vi "Write rotator.vi"(8 "error in (no error)":errorcluster, 10 "Rotator.lvclass":refnum<class "Rotator.lvclass">, 11 "ScienceTargetConfiguration in":refnum<class "ScienceTargetConfiguration.lvclass">) -> (0 "error out":errorcluster, 3 "ScienceTargetConfiguration out":refnum<class "ScienceTargetConfiguration.lvclass">)   [LabVIEW 2014, in "TCSDataDefinitions.lvlib" / "TCSCommand.lvlib" / "TargetConfiguration.lvlib" / "ScienceTargetConfiguration.lvclass"]
uses:
  ScienceTargetConfiguration.lvclass
  Rotator/Rotator.lvclass
  ScienceTargetConfiguration.lvclass/ScienceTargetConfiguration.ctl
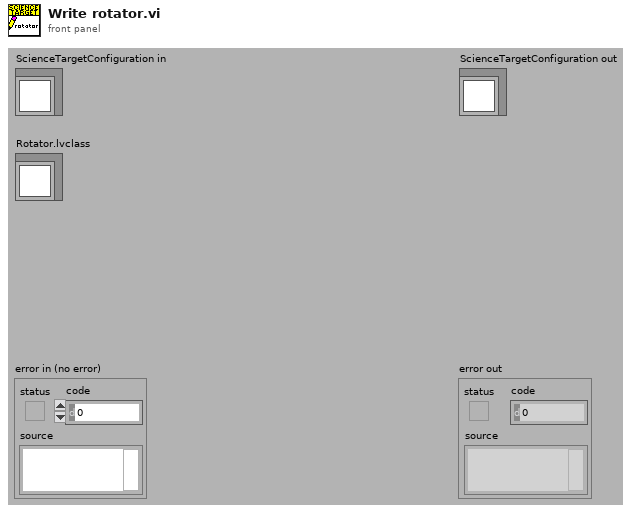
[diagram p1: front panel]
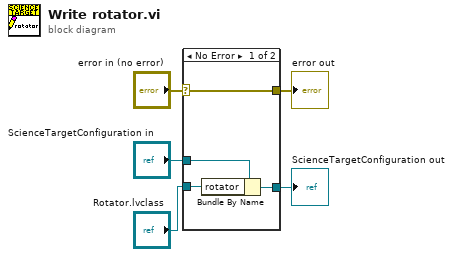
[diagram p0: block diagram]
diagram:
  n1 = case shown="No Error" "error in (no error)" {
    selector: "error in (no error)" -> [w9 w10]
    tunnel: [w9 w10] -> w4
    tunnel: [w7 w11] -> w2
    tunnel: "ScienceTargetConfiguration in" -> [w8 w11]
    tunnel: "Rotator.lvclass" -> [w6 _]
    frame No Error {
      n2 = Bundle By Name(cluster=w8, "rotator"=w6) -> (w7:refnum<class "ScienceTargetConfiguration.lvclass">)
    }
    frame Error {
    }
  }
  "error out" <- w4
  "ScienceTargetConfiguration out" <- w2
